vi "Lognormal PDF.vi"(9 "c":dbl=0.6, 10 "b":dbl=1.0, 11 "x":dbl=2.9999999999999973) -> (0 "error":i32, 3 "pdf(x)":dbl=0.04145929405577445)   [LabVIEW 2020, in "NI_Gmath.lvlib"]
doc: "Computes the continuous probability density function (PDF) of various distributions. You must manually select the polymorphic instance to use."
uses:
  NI_Gmath.lvlib
  st_error_code.ctl
panel:
  # "Lognormal PDF"
  # "median (scale)"
  # "standard dev (shape)"
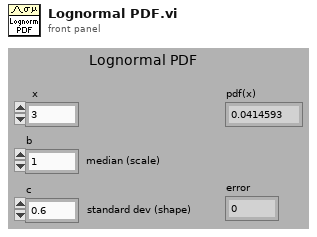
[diagram p1: front panel]
types:
  T1 = typedef "NI_Gmath.lvlib/st_error_code.ctl" = i32
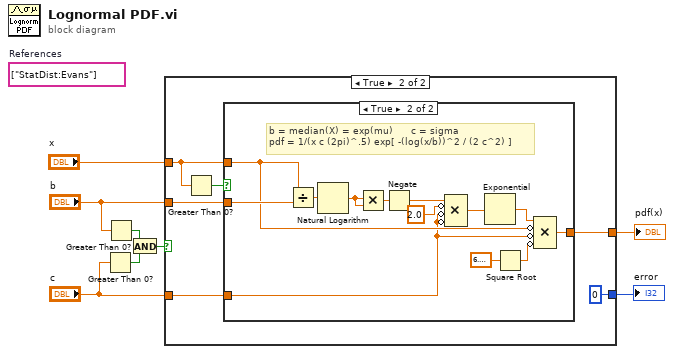
[diagram p0: block diagram]
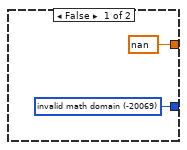
[diagram p2: hidden frame]
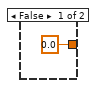
[diagram p3: hidden frame]
diagram:
  (unwired) string[] ["StatDist:Evans"]  # References
  n1 = Greater Than 0?(x="c") -> (x > 0?=w1:bool)
  n2 = Greater Than 0?(x="b") -> (x > 0?=w2:bool)
  n3 = And(x=w2, y=w1) -> (x .and. y?=w3:bool)
  n4 = case shown="True" w3 {
    tunnel: "c" -> [_ w13]
    tunnel: [w9 0 ("invalid math domain")] -> w8
    tunnel: [nan w14] -> w7
    tunnel: "x" -> [_ w11]
    tunnel: "b" -> [_ w15]
    frame False {
      w9 = T1 -20069 items=["invalid math domain"=-20069, "Fourier interpolation size m >= n"=-20070, "empty array"=-20003] ("stat interp error code")
    }
    frame True {
      n5 = Greater Than 0?(x=w11) -> (x > 0?=w12:bool)
      n6 = case shown="True" w12 {
        tunnel: w15 -> [_ w30]
        tunnel: [0.0 w29] -> w14
        tunnel: w11 -> [_ w24]
        tunnel: w13 -> [_ w19]
        frame False {
        }
        frame True {
          # "b = median(X) = exp(mu)      c = sigma\npdf = 1/(x c (2pi)^.5) exp[ -(log(x/b))^2 / (2 c^2) ]"
          n7 = Divide(x=w24, y=w30) -> (x/y=w27:dbl)
          n8 = Natural Logarithm(1:w27) -> (0:w26:dbl)
          n9 = Multiply(x=w26, y=w26) -> (x*y=w25:dbl)
          n10 = Negate(x=w25) -> (-x=w21:dbl)
          n11 = Compound Arithmetic op=MULTIPLY(w21, invert 2.0 ("value"), invert w19, invert w19) -> (w18:dbl)
          n12 = Exponential(1:w18) -> (0:w28:dbl)
          n13 = Square Root(x=6.283185307179586) -> (sqrt(x)=w22:dbl)
          n14 = Compound Arithmetic op=MULTIPLY(w28, invert w24, invert w19, invert w22) -> (w29:dbl)
        }
      }
    }
  }
  "pdf(x)" <- w7
  "error" <- w8
